vi "MR-Main.vi"() -> ()   [LabVIEW 2017]
doc: "The MyRIO MR-Main programme is a debug level operation that allows an authorised, TCP/IP capable controller to simulate customisable cooling events via control of a PWM servo and also transfer of information, including video, temperature and movement values.\nIf not connected to a remote controller, the programme will operate on a fix independent cooling cycle."
uses:
  <vilib>/myRIO/Express VI/Onboard Devices/Accelerometer/Accelerometer Express VI.xnode
  <vilib>/myRIO/Instrument Drivers/Onboard Devices/Accelerometer/vis/Read.vi
  <vilib>/myRIO/Instrument Drivers/Onboard Devices/Accelerometer/Accelerometer.lvlib
  <vilib>/myRIO/Common/Instrument Driver Framework/myRIO v1.0/Accelerometer/typedefs/Accelerometer Channels Enum.ctl
  <vilib>/myRIO/Common/Instrument Driver Framework/myRIO v1.0/Accelerometer/typedefs/Accelerometer Channels List.ctl
  <vilib>/myRIO/Common/Instrument Driver Framework/Utilities/typedefs/Generic FPGA Reference.ctl
  <vilib>/myRIO/Common/Instrument Driver Framework/Utilities/typedefs/myRIO v1.0 Reference.ctl
  <vilib>/myRIO/Common/Instrument Driver Framework/Utilities/typedefs/Hardware Version Enum.ctl
  <vilib>/myRIO/Common/Instrument Driver Framework/Utilities/typedefs/myRIO Generic Hardware Reference.ctl
  <vilib>/myRIO/Instrument Drivers/Onboard Devices/Accelerometer/typedefs/Accelerometer Reference.ctl
  <vilib>/myRIO/Instrument Drivers/Onboard Devices/Accelerometer/vis/myRIO Accelerometer Open.xnode
  <vilib>/myRIO/Common/Instrument Driver Framework/Utilities/vis/Is FPGA Ref Available.vi
  <vilib>/myRIO/Common/Instrument Driver Framework/myRIO v1.0/Accelerometer/vis/myRIO v1.1 Open Accelerometer.vi
  <vilib>/userdefined/High Color/nirio_resource_hc.ctl
  <vilib>/myRIO/Express VI/Onboard IO/AI/AI Express VI.xnode
  <vilib>/myRIO/Instrument Drivers/Onboard IO/AI/vis/Read.vi
  <vilib>/myRIO/Instrument Drivers/Onboard IO/AI/AI.lvlib
  <vilib>/myRIO/Common/Instrument Driver Framework/Utilities/typedefs/Analog Scaling Constants.ctl
  <vilib>/myRIO/Common/Instrument Driver Framework/Utilities/typedefs/Analog Scaling Constants List.ctl
  <vilib>/myRIO/Common/Instrument Driver Framework/myRIO v1.0/AI/typedefs/AI Channels Enum.ctl
  <vilib>/myRIO/Common/Instrument Driver Framework/myRIO v1.0/AI/typedefs/AI Channels List.ctl
  <vilib>/myRIO/Instrument Drivers/Onboard IO/AI/typedefs/AI Reference.ctl
  <vilib>/myRIO/Instrument Drivers/Onboard IO/AI/vis/myRIO AI Open.xnode
  <vilib>/myRIO/Common/Instrument Driver Framework/myRIO v1.0/AI/vis/myRIO v1.1 Open AI.vi
  <vilib>/myRIO/Express VI/Onboard Devices/LED/LED Express VI.xnode
  <vilib>/myRIO/Instrument Drivers/Onboard IO/DIO/vis/Write.vi
  <vilib>/myRIO/Instrument Drivers/Onboard IO/DIO/DIO.lvlib
  <vilib>/myRIO/Common/Instrument Driver Framework/myRIO v1.0/DIO/typedefs/DIO Channels Enum.ctl
  <vilib>/myRIO/Common/Instrument Driver Framework/myRIO v1.0/DIO/typedefs/DIO Channels List.ctl
  <vilib>/myRIO/Instrument Drivers/Onboard IO/DIO/typedefs/DIO Reference.ctl
  <vilib>/myRIO/Instrument Drivers/Onboard IO/DIO/vis/myRIO DIO Open.xnode
  <vilib>/myRIO/Common/Instrument Driver Framework/myRIO v1.0/DIO/vis/myRIO v1.1 Open DIO.vi
  <vilib>/myRIO/Express VI/Onboard IO/PWM/PWM Express VI.xnode
  <vilib>/myRIO/Instrument Drivers/Onboard IO/PWM/vis/Set Duty Cycle and Frequency.vi
  <vilib>/myRIO/Instrument Drivers/Onboard IO/PWM/PWM.lvlib
  <vilib>/myRIO/Instrument Drivers/Onboard IO/PWM/typedefs/PWM Configuration.ctl
  <vilib>/myRIO/Common/Instrument Driver Framework/myRIO v1.0/PWM/typedefs/PWM Channels Enum.ctl
  <vilib>/myRIO/Instrument Drivers/Onboard IO/PWM/typedefs/PWM Reference.ctl
  <vilib>/myRIO/Instrument Drivers/Onboard IO/PWM/vis/myRIO PWM Open.xnode
  <vilib>/myRIO/Common/Instrument Driver Framework/myRIO v1.0/PWM/vis/myRIO v1.1 Open PWM.vi
  <vilib>/myRIO/Express VI/Onboard Devices/Button/Button Express VI.xnode
  <vilib>/myRIO/Instrument Drivers/Onboard IO/DIO/vis/Read.vi
  <vilib>/myRIO/Instrument Drivers/Utilities/Utilities.lvlib
  <vilib>/vision/driver/NI_Vision_Acquisition_Software.lvlib
  <vilib>/userdefined/High Color/IMAQdx.ctl
  <resource>/objmgr/imaqdx.rc
panel:
  in  "Timeout Control":i32=30
  in  "Turn Off Counter":i32=10
  out "Turn Off Timer":timestamp format="%<%H:%M:%S>T"
  in  "Destruction Counter":i32=10
  in  "VideoMode":u32
  in  "Session In":T1
  out "Timeout":bool
  out "Timeout":timestamp format="%<%H:%M:%S>T"
  out "Scheduler":bool
  out "Destroyed":bool
  out "Destruction Timer":timestamp format="%<%H:%M:%S>T"
  in  "Disconnect":bool
  in  "Status Value":u8=1
  out "Local\nRequest":bool
  out "Movement\nDetected":bool
  out "Movement Event Array":bool[](array[boolean])
  in  "Lower\nTolerance":dbl=1.0 format="%#.3g"
  in  "Upper\nTolerance":dbl=1.0 format="%#.13g"
  out "Cooling Event Array":bool[](array[boolean])
  out "System Time":timestamp format="%<%H:%M:%S>T"
  in  "Cooling 4 Off":timestamp format="%<%H:%M:%S>T"
  in  "Cooling 4 On":timestamp format="%<%H:%M:%S>T"
  in  "Cooling 3 Off":timestamp format="%<%H:%M:%S>T"
  in  "Cooling 3 On":timestamp format="%<%H:%M:%S>T"
  in  "Cooling 2 Off":timestamp format="%<%H:%M:%S>T"
  in  "Cooling 2 On":timestamp format="%<%H:%M:%S>T"
  in  "Cooling 1 Off":timestamp format="%<%H:%M:%S>T"
  in  "Cooling 1 On":timestamp format="%<%H:%M:%S>T"
  out "Master Controller":bool
  out "Local Controller":bool
  out "Emergency Cooling":bool
  out "Initial Z":dbl=1.0 format="%#_13g"
  out "Initial Y":dbl=1.0 format="%#_13g"
  out "Initial X":dbl=1.0 format="%#_13g"
  in  "Emergency Temp (C)":u32=26
  out "source":string
  out "status":bool
  out "code":i32
  out "Net Error Code":i32
  out "Temp (C)":dbl format="%#.1g"
  out "Scheduled Cooling":bool
  out "Cooling 4":bool
  out "Cooling 3":bool
  out "Cooling 2":bool
  out "Cooling 1":bool
  out "Waveform Chart":T2(graph)
  out "String Length":i32
  out "Bytes Written":i32
  in  "Stop":bool
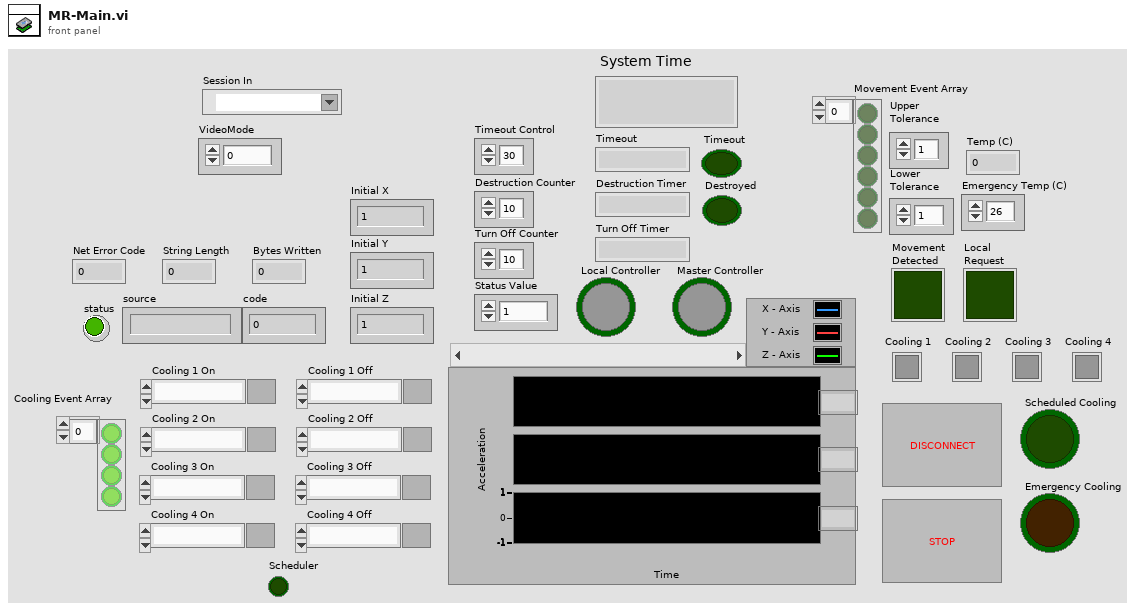
[diagram p1: front panel]
types:
  T1 = typedef "IMAQdx.ctl" = refnum<k21>
  T2 = cluster{"X-Axis":dbl, "Y-Axis":dbl, "Z-Axis":dbl}
  T3 = typedef "DIO.lvlib/DIO Reference.ctl" = cluster{"myRIO Reference":T4, "DIO Channels List":T8}
  T4 = typedef "myRIO Generic Hardware Reference.ctl" = cluster{"myRIO Model":T5, "myRIO Hardware Reference":T6}
  T5 = typedef "Hardware Version Enum.ctl" = enum16{"Unknown", "myRIO-1900", "myRIO-1950", "roboRIO", "NI ELVIS RIO CM"}
  T6 = typedef "myRIO v1.0 Reference.ctl" = cluster{"Generic FPGA Reference":T7, "Allow multiple opens":bool}
  T7 = typedef "Generic FPGA Reference.ctl" = refnum<k20>
  T8 = typedef "DIO Channels List.ctl" = T9[]
  T9 = typedef "DIO Channels Enum.ctl" = enum16{"Not Connected", "C/DIO0", "C/DIO1", "C/DIO2", "C/DIO3", "C/DIO4", "C/DIO5", "C/DIO6", "C/DIO7", "A/DIO0", "A/DIO1", "A/DIO2", "A/DIO3", "A/DIO4", "A/DIO5", "A/DIO6", "A/DIO7", "A/DIO8", "A/DIO9", "A/DIO10", "A/DIO11", "A/DIO12", "A/DIO13", "A/DIO14", "A/DIO15", "B/DIO0", "B/DIO1", "B/DIO2", "B/DIO3", "B/DIO4", "B/DIO5", "B/DIO6", "B/DIO7", "B/DIO8", "B/DIO9", "B/DIO10", "B/DIO11", "B/DIO12", "B/DIO13", "B/DIO14", "B/DIO15", "LED0", "LED1", "LED2", "LED3", "Button0", "DIO/DIO0", "DIO/DIO1", "DIO/DIO2", "DIO/DIO3", "DIO/DIO4", "DIO/DIO5", "DIO/DIO6", "DIO/DIO7", "DIO/DIO8", "DIO/DIO9", "SPI/CS0", "SPI/CS1", "SPI/CS2", "SPI/CS3", "LED RADIO (Green)", "LED RADIO (Red)", "LED COMM (Green)", "LED COMM (Red)", "LED MODE (Green)", "LED MODE (Red)"}
  T10 = typedef "nirio_resource_hc.ctl" = tag
  T11 = typedef "AI.lvlib/AI Reference.ctl" = cluster{"myRIO Reference":T4, "AI Channels List":T12, "AI Scaling Constants List":T14}
  T12 = typedef "AI Channels List.ctl" = T13[]
  T13 = typedef "AI Channels Enum.ctl" = enum16{"Not Connected", "AudioIn/Left", "AudioIn/Right", "C/AI0", "C/AI1", "A/AI0", "A/AI1", "A/AI2", "A/AI3", "B/AI0", "B/AI1", "B/AI2", "B/AI3", "AI/AI0", "AI/AI1", "AI/AI2", "AI/AI3"}
  T14 = typedef "Analog Scaling Constants List.ctl" = T15[]
  T15 = typedef "Analog Scaling Constants.ctl" = cluster{"LSB Weight (Volts)":dbl, "Offset (Volts)":dbl, "Signed?":bool}
  T16 = typedef "PWM.lvlib/PWM Reference.ctl" = cluster{"myRIO Reference":T4, "PWM Channels Enum":T17, "PWM Configuration":T18}
  T17 = typedef "PWM Channels Enum.ctl" = enum16{"Not Connected", "C/PWM0", "C/PWM1", "A/PWM0", "A/PWM1", "A/PWM2", "B/PWM0", "B/PWM1", "B/PWM2", "PWM/PWM0", "PWM/PWM1", "PWM/PWM2", "PWM/PWM3", "PWM/PWM4", "PWM/PWM5", "PWM/PWM6", "PWM/PWM7", "PWM/PWM8", "PWM/PWM9"}
  T18 = typedef "PWM.lvlib/PWM Configuration.ctl" = cluster{"Frequency":dbl, "Duty Cycle":dbl}
  T19 = typedef "Accelerometer.lvlib/Accelerometer Reference.ctl" = cluster{"myRIO Reference":T4, "Accelerometer Channels List":T20, "LSB Weight":dbl}
  T20 = typedef "Accelerometer Channels List.ctl" = T21[]
  T21 = typedef "Accelerometer Channels Enum.ctl" = enum16{"Not Connected", "X-Axis", "Y-Axis", "Z-Axis"}
  T22 = typedef "Image Type" = u32
  T23 = typedef "IMAQ Image.ctl" = refnum<image>
  T24 = cluster{dbl, dbl, dbl, dbl, bool, u8, "Status Value":u8}
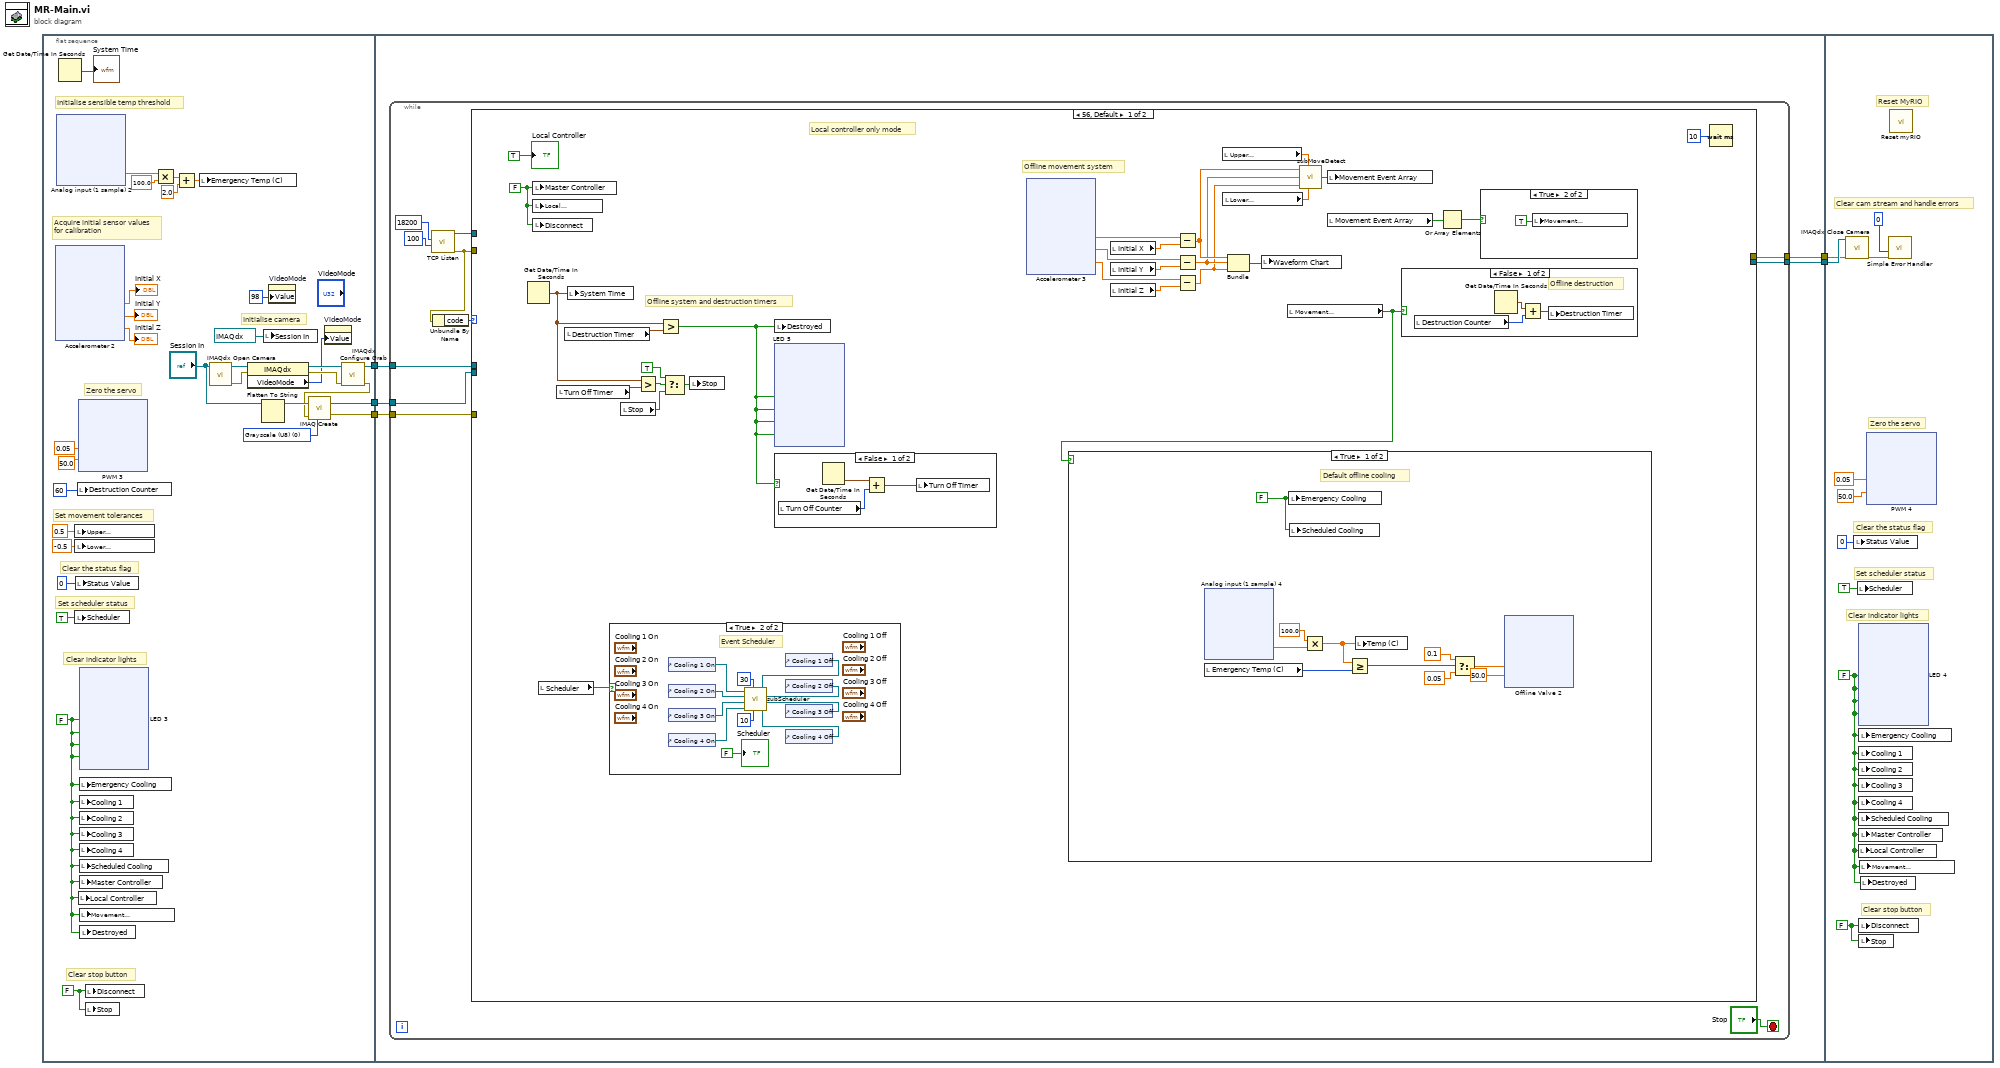
[diagram p0: block diagram]
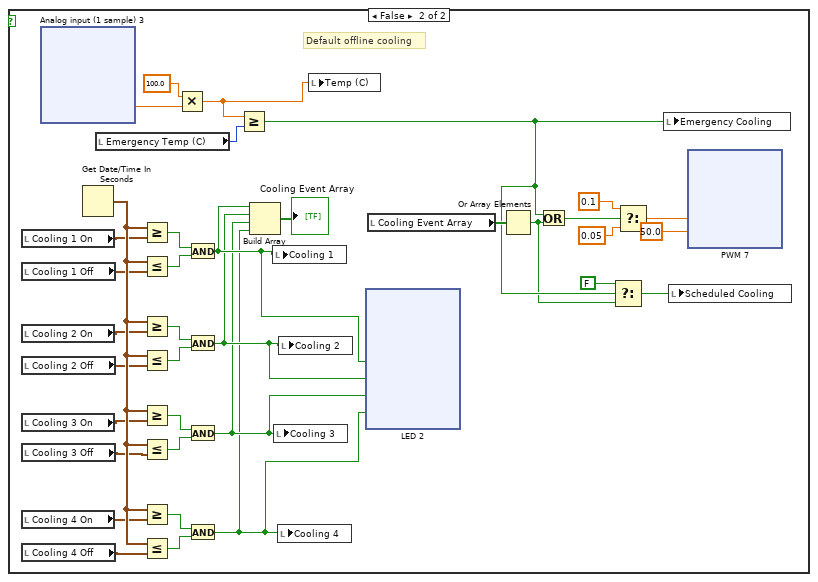
[diagram p3: hidden frame]
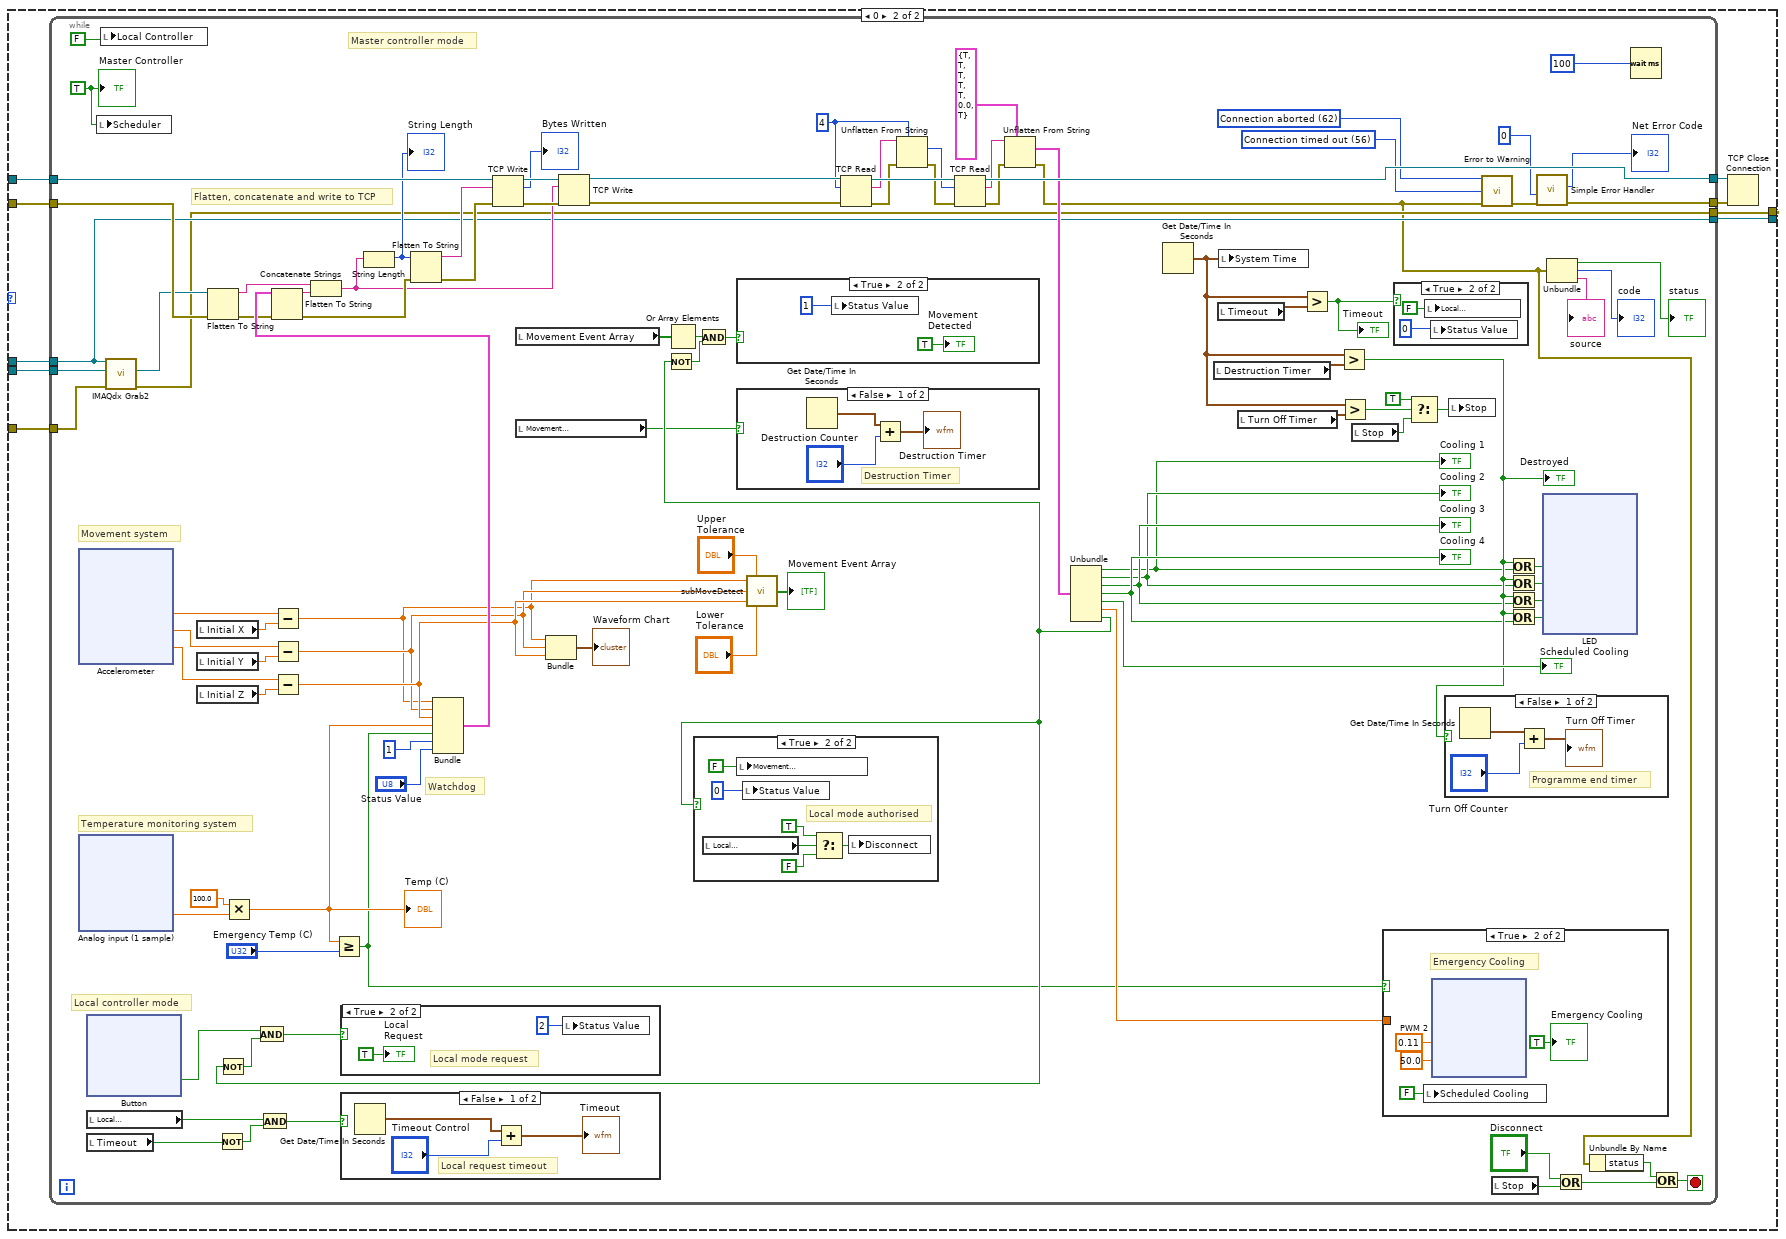
[diagram p7: hidden frame]
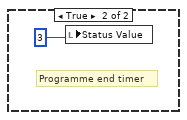
[diagram p8: hidden frame]
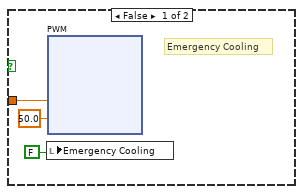
[diagram p15: hidden frame]
diagram:
  n1 = flat-sequence {
    tunnel: [w20] -> w5
    tunnel: [w19] -> w4
    tunnel: [w10] -> w1
    tunnel: w5 -> [w191]
    tunnel: w4 -> [w190]
    tunnel: [w189] -> w3
    tunnel: [w188] -> w2
    tunnel: w1 -> [w187]
    tunnel: w3 -> [w919]
    tunnel: w2 -> [w918]
    frame #0 {
      w16 = T22 0 items=["Grayscale (U8)", "Grayscale (I16)", "Grayscale (SGL)", "Complex (CSG)", "RGB (U32)", "HSL (U32)", "RGB (U64)", "Grayscale (U16)"] ("Image Type")
      w9 = FALSE
      w24 = FALSE
      # "Set scheduler status"
      # "Clear the status flag"
      # "Initialise camera"
      # "Clear indicator lights"
      # "Set movement tolerances"
      # "Zero the servo"
      # "Initialise sensible temp threshold"
      # "Acquire initial sensor values\nfor calibration"
      # "Clear stop button"
      n2 = xnode "Accelerometer 2"() -> ("X-Axis"=→"Initial X":dbl, "Y-Axis"=→"Initial Y":dbl, "Z-Axis"=→"Initial Z":dbl)  [unwired: 1 in, 1 out]
      n3 = xnode "Analog input (1 sample) 2"() -> ("A/AI3 (Pin 9)"=w29:dbl)  [unwired: 1 in, 1 out]
      n4 = Get Date/Time In Seconds() -> (seconds since 1Jan1904=→"System Time":timestamp)
      n5 = local write "Upper\nTolerance"(0.5 ("Upper\nTolerance")) -> ()
      n6 = local write "Lower\nTolerance"(-0.5 ("Lower\nTolerance 2")) -> ()
      n7 = local write "Scheduler"(TRUE) -> ()
      n8 = local write "Status Value"(u8 0 ("Request Value")) -> ()
      n9 = local write "Destruction Counter"(60) -> ()
      n10 = xnode "PWM 3"("Duty Cycle"=0.05, "Frequency [Hz]"=50.0) -> ()  [unwired: 1 in, 1 out]
      n11 = local write "Local Controller"(w9) -> ()
      n12 = xnode "LED 3"("LED0"=w9, "LED1"=w9, "LED2"=w9, "LED3"=w9) -> ()  [unwired: 1 in, 1 out]
      n13 = local write "Emergency Cooling"(w9) -> ()
      n14 = local write "Cooling 1"(w9) -> ()
      n15 = local write "Cooling 2"(w9) -> ()
      n16 = local write "Cooling 3"(w9) -> ()
      n17 = local write "Cooling 4"(w9) -> ()
      n18 = local write "Scheduled Cooling"(w9) -> ()
      n19 = local write "Master Controller"(w9) -> ()
      n20 = local write "Movement\nDetected"(w9) -> ()
      n21 = local write "Destroyed"(w9) -> ()
      n22 = local write "Disconnect"(w24) -> ()
      n23 = local write "Stop"(w24) -> ()
      n24 = Multiply(x=w29, y=100.0) -> (x*y=w30:dbl)
      n25 = Add(x=w30, y=2.0) -> (x+y=w31:dbl)
      n26 = local write "Emergency Temp (C)"(w31) -> ()
      n27 = call <vilib>:"IMAQdx Open Camera.vi"("Session In"="Session In") -> ("error out"=w13:errorcluster, "Session Out"=w15:T1)  [unwired: 2 in, 7 out]
      n28 = property class="IMAQdx"(reference=w15, error in=w13) -> (reference out=w14:T1, error out=w12:errorcluster, "VideoMode"=w8:u32)
      n29 = Flatten To String(anything="Session In") -> (data string=w17:string)  [unwired: 3 in, 2 out]
      n30 = local write "Session In"(T1 "cam0" ("Session In")) -> ()
      n31 = property on="VideoMode" class="DigNum (strict)"("Value"=u32 98 ("VideoMode")) -> ()  [unwired: 2 in, 2 out]
      n32 = property on="VideoMode" class="DigNum (strict)"("Value"=w8) -> ()  [unwired: 2 in, 2 out]
      n33 = call <vilib>:"IMAQdx Configure Grab.vi"("error in"=w12, "Session In"=w14) -> ("error out"=w11:errorcluster, "Session Out"=w20:T1)  [unwired: 2 in, 6 out]
      n34 = call "IMAQ Create"("Image Name"=w17, "Image Type"=w16, "error in (no error)"=w11) -> ("New Image"=w19:T23, "error out"=w10:errorcluster)  [unwired: 2 in]
    }
    frame #1 {
      n35 = while {
        tunnel: w191 -> [w196]
        tunnel: w190 -> [w195]
        tunnel: [w194] -> w189
        tunnel: [w193] -> w188
        tunnel: w187 -> [w192]
        stop <- "Stop" stop-if-true
        n36 = call <vilib>:"TCP Listen.vi"("timeout ms (wait forever: -1)"=100, "port"=u16 18200 ("timeout ms (wait forever: -1)")) -> ("error out"=w198:errorcluster, "connection ID"=w201:refnum<k5>)  [unwired: 2 in, 6 out]
        n37 = Unbundle By Name(w198) -> ("code"=w197:i32)
        n38 = case shown="56, Default" w197 {
          tunnel: w201 -> [_ w562]
          tunnel: w198 -> [_ w561]
          tunnel: w196 -> [_ w558]
          tunnel: w195 -> [_ w557]
          tunnel: [_ w556] -> w194
          tunnel: [_ w555] -> w193
          tunnel: w192 -> [_ w554]
          frame 56, Default {
            w223 = FALSE
            # "Offline system and destruction timers"
            # "Offline movement system"
            # "Local controller only mode"
            n39 = Get Date/Time In Seconds() -> (seconds since 1Jan1904=w208:timestamp)
            n40 = local write "Master Controller"(w223) -> ()
            n41 = local write "Local\nRequest"(w223) -> ()
            n42 = local write "Disconnect"(w223) -> ()
            n43 = local read "Scheduler"() -> (w212:bool)
            n44 = local read "Turn Off Timer"() -> (w209:timestamp)
            n45 = local read "Destruction Timer"() -> (w214:timestamp)
            n46 = local write "System Time"(w208) -> ()
            n47 = case shown="True" w212 {
              frame False {
              }
              frame True {
                # "Event Scheduler"
                n48 = control-ref of="Cooling 1 On"() -> (w503:refnum<vi>)
                n49 = control-ref of="Cooling 2 On"() -> (w502:refnum<vi>)
                n50 = control-ref of="Cooling 3 On"() -> (w501:refnum<vi>)
                n51 = control-ref of="Cooling 4 On"() -> (w500:refnum<vi>)
                n52 = control-ref of="Cooling 1 Off"() -> (w507:refnum<vi>)
                n53 = control-ref of="Cooling 2 Off"() -> (w505:refnum<vi>)
                n54 = control-ref of="Cooling 3 Off"() -> (w504:refnum<vi>)
                n55 = control-ref of="Cooling 4 Off"() -> (w506:refnum<vi>)
                n56 = call "subScheduler.vi"("Cooling 4 Off"=w506, "Cooling 3 Off"=w504, "Cooling 2 Off"=w505, "Cooling 1 Off"=w507, "Deactivate Offset"=10, "Activate Offset"=30, "Cooling 4 On"=w500, "Cooling 3 On"=w501, "Cooling 2 On"=w502, "Cooling 1 On"=w503) -> ()
                "Scheduler" <- FALSE
              }
            }
            n57 = local read "Stop"() -> (w204:bool)
            n58 = Greater?(x=w208, y=w209) -> (0:w206:bool)
            n59 = Greater?(x=w208, y=w214) -> (0:w207:bool)
            n60 = Select(t=TRUE, s=w206, f=w204) -> (s? t:f=w205:bool)
            n61 = local write "Stop"(w205) -> ()
            n62 = case shown="False" w207 {
              frame False {
                n63 = local read "Turn Off Counter"() -> (w232:i32)
                n64 = Get Date/Time In Seconds() -> (seconds since 1Jan1904=w233:timestamp)
                n65 = Add(x=w233, y=w232) -> (x+y=w231:timestamp)
                n66 = local write "Turn Off Timer"(w231) -> ()
              }
              frame True {
              }
            }
            n67 = local write "Destroyed"(w207) -> ()
            n68 = xnode "LED 5"("LED0"=w207, "LED1"=w207, "LED2"=w207, "LED3"=w207) -> ()  [unwired: 1 in, 1 out]
            n69 = xnode "Accelerometer 3"() -> ("X-Axis"=w226:dbl, "Y-Axis"=w228:dbl, "Z-Axis"=w230:dbl)  [unwired: 1 in, 1 out]
            n70 = local read "Initial X"() -> (w225:dbl)
            n71 = local read "Initial Y"() -> (w227:dbl)
            n72 = local read "Initial Z"() -> (w229:dbl)
            n73 = Subtract(x=w226, y=w225) -> (x-y=w221:dbl)
            n74 = Subtract(x=w228, y=w227) -> (x-y=w220:dbl)
            n75 = Subtract(x=w230, y=w229) -> (x-y=w219:dbl)
            n76 = local read "Upper\nTolerance"() -> (w217:dbl)
            n77 = local read "Lower\nTolerance"() -> (w218:dbl)
            n78 = Bundle(w221, w220, w219) -> (w224:cluster{dbl, dbl, dbl})  [unwired: 1 in]
            n79 = local write "Waveform Chart"(w224) -> ()
            n80 = local read "Movement\nDetected"() -> (w211:bool)
            n81 = case shown="True" w211 {
              frame True {
                w281 = FALSE
                # "Default offline cooling"
                n82 = xnode "Analog input (1 sample) 4"() -> ("A/AI3 (Pin 9)"=w276:dbl)  [unwired: 1 in, 1 out]
                n83 = local read "Emergency Temp (C)"() -> (w274:u32)
                n84 = local write "Emergency Cooling"(w281) -> ()
                n85 = local write "Scheduled Cooling"(w281) -> ()
                n86 = Multiply(x=100.0, y=w276) -> (x*y=w273:dbl)
                n87 = Greater Or Equal?(x=w273, y=w274) -> (x >= y?=w272:bool)
                n88 = local write "Temp (C)"(w273) -> ()
                n89 = Select(t=0.1, s=w272, f=0.05) -> (s? t:f=w277:dbl)
                n90 = xnode "Offline Valve 2"("Duty Cycle"=w277, "Frequency [Hz]"=50.0) -> ()  [unwired: 1 in, 1 out]
              }
              frame False {
                # "Default offline cooling"
                n91 = local read "Cooling 1 On"() -> (w380:timestamp)
                n92 = local read "Cooling 1 Off"() -> (w379:timestamp)
                n93 = local read "Cooling 2 On"() -> (w378:timestamp)
                n94 = local read "Cooling 2 Off"() -> (w377:timestamp)
                n95 = local read "Cooling 3 On"() -> (w376:timestamp)
                n96 = local read "Cooling 3 Off"() -> (w375:timestamp)
                n97 = local read "Cooling 4 On"() -> (w374:timestamp)
                n98 = local read "Cooling 4 Off"() -> (w373:timestamp)
                n99 = xnode "Analog input (1 sample) 3"() -> ("A/AI3 (Pin 9)"=w364:dbl)  [unwired: 1 in, 1 out]
                n100 = Get Date/Time In Seconds() -> (seconds since 1Jan1904=w381:timestamp)
                n101 = local read "Emergency Temp (C)"() -> (w363:u32)
                n102 = Greater Or Equal?(x=w381, y=w380) -> (x >= y?=w388:bool)
                n103 = Less Or Equal?(x=w381, y=w379) -> (x <= y?=w389:bool)
                n104 = Greater Or Equal?(x=w381, y=w378) -> (x >= y?=w387:bool)
                n105 = Less Or Equal?(x=w381, y=w377) -> (x <= y?=w386:bool)
                n106 = Greater Or Equal?(x=w381, y=w376) -> (x >= y?=w384:bool)
                n107 = Less Or Equal?(x=w381, y=w375) -> (x <= y?=w385:bool)
                n108 = Greater Or Equal?(x=w381, y=w374) -> (x >= y?=w383:bool)
                n109 = Less Or Equal?(x=w381, y=w373) -> (x <= y?=w382:bool)
                n110 = Multiply(x=100.0, y=w364) -> (x*y=w362:dbl)
                n111 = And(x=w388, y=w389) -> (x .and. y?=w369:bool)
                n112 = And(x=w387, y=w386) -> (x .and. y?=w368:bool)
                n113 = And(x=w384, y=w385) -> (x .and. y?=w367:bool)
                n114 = And(x=w383, y=w382) -> (x .and. y?=w366:bool)
                n115 = Greater Or Equal?(x=w362, y=w363) -> (x >= y?=w359:bool)
                n116 = Build Array(w369, w368, w367, w366) -> (→"Cooling Event Array":bool[])
                n117 = local write "Cooling 1"(w369) -> ()
                n118 = local write "Cooling 3"(w367) -> ()
                n119 = local write "Cooling 4"(w366) -> ()
                n120 = local write "Cooling 2"(w368) -> ()
                n121 = local write "Temp (C)"(w362) -> ()
                n122 = xnode "LED 2"("LED0"=w369, "LED1"=w368, "LED2"=w367, "LED3"=w366) -> ()  [unwired: 1 in, 1 out]
                n123 = local read "Cooling Event Array"() -> (w371:bool[])
                n124 = Or Array Elements(Boolean array=w371) -> (logical OR=w358:bool)
                n125 = Or(x=w359, y=w358) -> (x .or. y?=w361:bool)
                n126 = Select(t=FALSE, s=w359, f=w358) -> (s? t:f=w356:bool)
                n127 = Select(t=0.1, s=w361, f=0.05) -> (s? t:f=w354:dbl)
                n128 = local write "Emergency Cooling"(w359) -> ()
                n129 = local write "Scheduled Cooling"(w356) -> ()
                n130 = xnode "PWM 7"("Duty Cycle"=w354, "Frequency [Hz]"=50.0) -> ()  [unwired: 1 in, 1 out]
              }
            }
            n131 = call "subMoveDetect.vi"("X"=w221, "Upper\nTolerance"=w217, "Y"=w220, "Z"=w219, "Lower\nTolerance"=w218) -> ("Movement Event Array"=w222:bool[])
            n132 = local write "Movement Event Array"(w222) -> ()
            n133 = local read "Movement Event Array"() -> (w216:bool[])
            n134 = case shown="False" w211 {
              frame False {
                # "Offline destruction"
                n135 = local read "Destruction Counter"() -> (w512:i32)
                n136 = Get Date/Time In Seconds() -> (seconds since 1Jan1904=w514:timestamp)
                n137 = Add(x=w514, y=w512) -> (x+y=w513:timestamp)
                n138 = local write "Destruction Timer"(w513) -> ()
              }
              frame True {
              }
            }
            n139 = Or Array Elements(Boolean array=w216) -> (logical OR=w215:bool)
            n140 = case shown="True" w215 {
              frame False {
              }
              frame True {
                n141 = local write "Movement\nDetected"(TRUE) -> ()
              }
            }
            n142 = Wait (ms)(milliseconds to wait=u32 10) -> ()  [unwired: 1 out]
            "Local Controller" <- TRUE
          }
          frame 0 {
            n143 = while {
              tunnel: w562 -> [w662]
              tunnel: w561 -> [w581]
              tunnel: [w604] -> w560
              tunnel: [w656] -> w559
              tunnel: w558 -> [w578]
              tunnel: w557 -> [w579]
              tunnel: [w578] -> w556
              tunnel: [w573] -> w555
              tunnel: w554 -> [w577]
              stop <- w661 stop-if-true
              w592 = TRUE
              w650 = 56 items=["No Error", "Argument Error", "Memory Full", "Out of Zone", "End of File", "File Already Open", "Generic File IO Error", "File Not Found", "File Permission Error", "Disk Full", "Duplicate Path", "Too Many Files Open", "Not Enabled", "Resource File Not Found", "Cannot Add Resource", "Resource Not Found", "Image Not Found", "Image Memory Error", "Pen Does Not Exist", "Config Bad Type", "Config Token Not Found", "Config Parse Error", "Config Memory Error", "Bad External Code Format", "Bad External Code Offset", "External Code Not Present", "Null Window", "Destroy Window Mixup", "Null Menu", "Print Aborted", "Bad Print Record", "Print Driver Error", "Windows Error During Print", "Memory Error During Print", "Print Dialog Error", "Generic Print Error", "Invalid Device Refnum", "Device Not Found", "Device Parameter Error", "Device Unit Error", "Can't Open Device", "Device Call Aborted", "Generic Error", "Cancelled By User", "Object ID Too Low", "Object ID Too High", "Object Not In Heap", "Unknown Heap", "Bad DefProc ID", "DefProc Not In Table", "Message Out Of Range", "Null Method", "Unknown Message", "Manager Call Not Supported", "Bad address", "Connection In progress", "Connection timed out", "Connection is already in progress", "Network attribute not supported", "Network error", "Address in use", "System out of memory", "Connection aborted", "Connection refused", "Connection is not connected", "Connection is already connected", "Connection closed", "Initialize error (interapplication manager)", "Bad occurrence", "Wait on unbound occurrence handler", "Occurrence queue overflow", "Bad path", "Semaphore not signaled", "Unrecognized type (interapplication manager)"] ("3rd Error to Convert")
              w651 = 62 items=["No Error", "Argument Error", "Memory Full", "Out of Zone", "End of File", "File Already Open", "Generic File IO Error", "File Not Found", "File Permission Error", "Disk Full", "Duplicate Path", "Too Many Files Open", "Not Enabled", "Resource File Not Found", "Cannot Add Resource", "Resource Not Found", "Image Not Found", "Image Memory Error", "Pen Does Not Exist", "Config Bad Type", "Config Token Not Found", "Config Parse Error", "Config Memory Error", "Bad External Code Format", "Bad External Code Offset", "External Code Not Present", "Null Window", "Destroy Window Mixup", "Null Menu", "Print Aborted", "Bad Print Record", "Print Driver Error", "Windows Error During Print", "Memory Error During Print", "Print Dialog Error", "Generic Print Error", "Invalid Device Refnum", "Device Not Found", "Device Parameter Error", "Device Unit Error", "Can't Open Device", "Device Call Aborted", "Generic Error", "Cancelled By User", "Object ID Too Low", "Object ID Too High", "Object Not In Heap", "Unknown Heap", "Bad DefProc ID", "DefProc Not In Table", "Message Out Of Range", "Null Method", "Unknown Message", "Manager Call Not Supported", "Bad address", "Connection In progress", "Connection timed out", "Connection is already in progress", "Network attribute not supported", "Network error", "Address in use", "System out of memory", "Connection aborted", "Connection refused", "Connection is not connected", "Connection is already connected", "Connection closed", "Initialize error (interapplication manager)", "Bad occurrence", "Wait on unbound occurrence handler", "Occurrence queue overflow", "Bad path", "Semaphore not signaled", "Unrecognized type (interapplication manager)"] ("1st Error to Convert")
              w630 = 4 ("bytes to read")
              # "Master controller mode"
              # "Movement system"
              # "Temperature monitoring system"
              # "Watchdog"
              # "Flatten, concatenate and write to TCP"
              # "Local controller mode"
              n144 = xnode "Accelerometer"() -> ("X-Axis"=w640:dbl, "Y-Axis"=w641:dbl, "Z-Axis"=w653:dbl)  [unwired: 1 in, 1 out]
              n145 = xnode "Analog input (1 sample)"() -> ("A/AI3 (Pin 9)"=w660:dbl)  [unwired: 1 in, 1 out]
              n146 = xnode "Button"() -> ("Value"=w611:bool)  [unwired: 1 in, 1 out]
              n147 = local read "Local\nRequest"() -> (w586:bool)
              n148 = local read "Timeout"() -> (w583:bool)
              n149 = local write "Scheduler"(w592) -> ()
              n150 = local write "Local Controller"(FALSE) -> ()
              n151 = call <vilib>:"IMAQdx Grab2.vi"("error in"=w577, "Image In"=w579, "Session In"=w578) -> ("error out"=w573:errorcluster, "Image Out"=w580:T23)  [unwired: 5 in, 2 out]
              n152 = local read "Initial X"() -> (w637:dbl)
              n153 = local read "Initial Y"() -> (w638:dbl)
              n154 = local read "Initial Z"() -> (w639:dbl)
              n155 = Flatten To String(anything=w580, error in (no error)=w581) -> (data string=w617:string, error out=w625:errorcluster)  [unwired: 2 in, 1 out]
              n156 = Not(x=w583) -> (.not. x?=w585:bool)
              n157 = Multiply(x=100.0, y=w660) -> (x*y=w649:dbl)
              "Temp (C)" <- w649
              n158 = And(x=w586, y=w585) -> (x .and. y?=w584:bool)
              n159 = Subtract(x=w640, y=w637) -> (x-y=w596:dbl)
              n160 = Subtract(x=w641, y=w638) -> (x-y=w597:dbl)
              n161 = Subtract(x=w653, y=w639) -> (x-y=w598:dbl)
              n162 = Greater Or Equal?(x=w649, y="Emergency Temp (C)") -> (x >= y?=w603:bool)
              n163 = case shown="False" w584 {
                frame False {
                  # "Local request timeout"
                  n164 = Get Date/Time In Seconds() -> (seconds since 1Jan1904=w673:timestamp)
                  n165 = Add(x=w673, y="Timeout Control") -> (x+y=→"Timeout":timestamp)
                }
                frame True {
                  # "Local request timeout"
                }
              }
              n166 = Bundle(w596, w597, w598, w649, w603, u8 1, "Status Value"="Status Value") -> (w634:T24)  [unwired: 1 in]
              n167 = Flatten To String(anything=w634, error in (no error)=w625) -> (data string=w619:string, error out=w624:errorcluster)  [unwired: 2 in, 1 out]
              n168 = Concatenate Strings(w617, w619) -> (w618:string)
              n169 = String Length(string=w618) -> (length=w633:i32)
              "String Length" <- w633
              n170 = Flatten To String(anything=w633, error in (no error)=w624) -> (data string=w632:string, error out=w623:errorcluster)  [unwired: 2 in, 1 out]
              n171 = TCP Write(connection ID=w662, data in=w632, error in (no error)=w623) -> (connection ID out=w663:refnum<k5>, bytes written=→"Bytes Written":i32, error out=w664:errorcluster)  [unwired: 1 out]
              n172 = local read "Movement Event Array"() -> (w635:bool[])
              n173 = local read "Movement\nDetected"() -> (w599:bool)
              n174 = Bundle(w596, w597, w598) -> (→"Waveform Chart":cluster{dbl, dbl, dbl})  [unwired: 1 in]
              n175 = TCP Write(connection ID=w663, data in=w618, error in (no error)=w664) -> (connection ID out=w658:refnum<k5>, error out=w643:errorcluster)  [unwired: 2 out]
              n176 = Or Array Elements(Boolean array=w635) -> (logical OR=w615:bool)
              n177 = case shown="False" w599 {
                frame False {
                  # "Destruction Timer"
                  n178 = Get Date/Time In Seconds() -> (seconds since 1Jan1904=w677:timestamp)
                  n179 = Add(x=w677, y="Destruction Counter") -> (x+y=→"Destruction Timer":timestamp)
                }
                frame True {
                }
              }
              n180 = call "subMoveDetect.vi"("X"=w596, "Upper\nTolerance"="Upper\nTolerance", "Y"=w597, "Z"=w598, "Lower\nTolerance"="Lower\nTolerance") -> ("Movement Event Array"=→"Movement Event Array":bool[])
              n181 = TCP Read(connection ID=w658, bytes to read=w630, error in (no error)=w643) -> (connection ID out=w657:refnum<k5>, data out=w631:string, error out=w622:errorcluster)  [unwired: 2 out]
              n182 = Unflatten From String(type=w630, binary string=w631, error in (no error)=w622) -> (value=w629:i32, error out=w621:errorcluster)  [unwired: 2 in, 1 out]
              n183 = TCP Read(connection ID=w657, bytes to read=w629, error in (no error)=w621) -> (connection ID out=w656:refnum<k5>, data out=w628:string, error out=w620:errorcluster)  [unwired: 2 out]
              n184 = Unflatten From String(type=cluster{bool, bool, bool, bool, bool, dbl, bool} {TRUE, TRUE, TRUE, TRUE, TRUE, 0.0, TRUE} ("Cluster"), binary string=w628, error in (no error)=w620) -> (value=w627:cluster{bool, bool, bool, bool, bool, dbl, bool}, error out=w567:errorcluster)  [unwired: 2 in, 1 out]
              n185 = Unbundle(w627) -> (w563:bool, w564:bool, w565:bool, w566:bool, →"Scheduled Cooling":bool, w644:dbl, w608:bool)
              "Cooling 1" <- w563
              "Cooling 2" <- w564
              "Cooling 3" <- w565
              "Cooling 4" <- w566
              n186 = Not(x=w608) -> (.not. x?=w612:bool)
              n187 = And(x=w611, y=w612) -> (x .and. y?=w613:bool)
              n188 = case shown="True" w613 {
                frame False {
                  # "Local mode request"
                }
                frame True {
                  # "Local mode request"
                  n189 = local write "Status Value"(u8 2 ("Request Value")) -> ()
                  "Local\nRequest" <- TRUE
                }
              }
              n190 = Not(x=w608) -> (.not. x?=w614:bool)
              n191 = case shown="True" w608 {
                frame False {
                }
                frame True {
                  # "Local mode authorised"
                  n192 = local read "Local\nRequest"() -> (w683:bool)
                  n193 = local write "Movement\nDetected"(FALSE) -> ()
                  n194 = local write "Status Value"(u8 0 ("Request Value")) -> ()
                  n195 = Select(t=TRUE, s=w683, f=FALSE) -> (s? t:f=w680:bool)
                  n196 = local write "Disconnect"(w680) -> ()
                }
              }
              n197 = And(x=w615, y=w614) -> (x .and. y?=w616:bool)
              n198 = case shown="True" w616 {
                frame False {
                }
                frame True {
                  n199 = local write "Status Value"(u8 1 ("Request Value")) -> ()
                  "Movement\nDetected" <- TRUE
                }
              }
              n200 = Get Date/Time In Seconds() -> (seconds since 1Jan1904=w568:timestamp)
              n201 = local read "Destruction Timer"() -> (w600:timestamp)
              n202 = local read "Timeout"() -> (w587:timestamp)
              n203 = local write "System Time"(w568) -> ()
              n204 = local read "Turn Off Timer"() -> (w575:timestamp)
              n205 = Greater?(x=w568, y=w587) -> (0:w582:bool)
              "Timeout" <- w582
              n206 = Greater?(x=w568, y=w600) -> (0:w576:bool)
              "Destroyed" <- w576
              n207 = Greater?(x=w568, y=w575) -> (0:w572:bool)
              n208 = local read "Stop"() -> (w570:bool)
              n209 = case shown="True" w603 {
                tunnel: w644 -> [w690 _]
                frame False {
                  # "Emergency Cooling"
                  n210 = local write "Emergency Cooling"(FALSE) -> ()
                  n211 = xnode "PWM"("Duty Cycle"=w690, "Frequency [Hz]"=50.0) -> ()  [unwired: 1 in, 1 out]
                }
                frame True {
                  # "Emergency Cooling"
                  n212 = local write "Scheduled Cooling"(FALSE) -> ()
                  n213 = xnode "PWM 2"("Duty Cycle"=0.11, "Frequency [Hz]"=50.0) -> ()  [unwired: 1 in, 1 out]
                  "Emergency Cooling" <- TRUE
                }
              }
              n214 = case shown="True" w582 {
                frame False {
                }
                frame True {
                  n215 = local write "Local\nRequest"(FALSE) -> ()
                  n216 = local write "Status Value"(u8 0 ("Request Value")) -> ()
                }
              }
              n217 = Select(t=TRUE, s=w572, f=w570) -> (s? t:f=w569:bool)
              n218 = case shown="False" w576 {
                frame False {
                  # "Programme end timer"
                  n219 = Get Date/Time In Seconds() -> (seconds since 1Jan1904=w668:timestamp)
                  n220 = Add(x=w668, y="Turn Off Counter") -> (x+y=→"Turn Off Timer":timestamp)
                }
                frame True {
                  # "Programme end timer"
                  n221 = local write "Status Value"(u8 3 ("Request Value")) -> ()
                }
              }
              n222 = local write "Stop"(w569) -> ()
              n223 = call <vilib>:"Error to Warning.vi"("1st Error to Convert"=w651, "3rd Error to Convert"=w650, "error in"=w567) -> ("warning out"=w602:errorcluster)  [unwired: 3 in, 9 out]
              n224 = local read "Stop"() -> (w606:bool)
              n225 = Or(x=w576, y=w563) -> (x .or. y?=w591:bool)
              n226 = Or(x=w576, y=w564) -> (x .or. y?=w590:bool)
              n227 = Or(x=w576, y=w565) -> (x .or. y?=w589:bool)
              n228 = Or(x=w576, y=w566) -> (x .or. y?=w588:bool)
              n229 = call <vilib>:"Simple Error Handler.vi"("type of dialog (OK msg:1)"=0, "error in (no error)"=w602) -> ("code out"=→"Net Error Code":i32, "error out"=w604:errorcluster)  [unwired: 6 out]
              n230 = xnode "LED"("LED0"=w591, "LED1"=w590, "LED2"=w589, "LED3"=w588) -> ()  [unwired: 1 in, 1 out]
              n231 = Unbundle(w567) -> ("status"=→"status":bool, "code"=→"code":i32, "source"=→"source":string)
              n232 = Or(x="Disconnect", y=w606) -> (x .or. y?=w605:bool)
              n233 = Unbundle By Name(w567) -> ("status"=w642:bool)
              n234 = Wait (ms)(milliseconds to wait=u32 100) -> ()  [unwired: 1 out]
              n235 = Or(x=w642, y=w605) -> (x .or. y?=w661:bool)
              "Master Controller" <- w592
            }
            n236 = TCP Close Connection(connection ID=w559, error in (no error)=w560) -> ()  [unwired: 3 out]
          }
        }
      }
    }
    frame #2 {
      w917 = FALSE
      w914 = FALSE
      # "Clear cam stream and handle errors"
      # "Set scheduler status"
      # "Clear the status flag"
      # "Clear indicator lights"
      # "Zero the servo"
      # "Reset MyRIO"
      # "Clear stop button"
      n237 = call <vilib>:"IMAQdx Close Camera.vi"("error in"=w918, "Session In"=w919) -> ("error out"=w916:errorcluster)  [unwired: 9 in]
      n238 = local write "Status Value"(u8 0 ("Request Value")) -> ()
      n239 = local write "Scheduler"(TRUE) -> ()
      n240 = local write "Local Controller"(w917) -> ()
      n241 = xnode "LED 4"("LED0"=w917, "LED1"=w917, "LED2"=w917, "LED3"=w917) -> ()  [unwired: 1 in, 1 out]
      n242 = local write "Emergency Cooling"(w917) -> ()
      n243 = local write "Cooling 1"(w917) -> ()
      n244 = local write "Cooling 2"(w917) -> ()
      n245 = local write "Cooling 3"(w917) -> ()
      n246 = local write "Cooling 4"(w917) -> ()
      n247 = local write "Scheduled Cooling"(w917) -> ()
      n248 = local write "Master Controller"(w917) -> ()
      n249 = local write "Disconnect"(w914) -> ()
      n250 = local write "Stop"(w914) -> ()
      n251 = local write "Movement\nDetected"(w917) -> ()
      n252 = local write "Destroyed"(w917) -> ()
      n253 = xnode "PWM 4"("Duty Cycle"=0.05, "Frequency [Hz]"=50.0) -> ()  [unwired: 1 in, 1 out]
      n254 = call <vilib>:"Simple Error Handler.vi"("type of dialog (OK msg:1)"=0, "error in (no error)"=w916) -> ()  [unwired: 8 out]
      n255 = call <vilib>:"Reset myRIO.vi"() -> ()  [unwired: 11 in, 1 out]
    }
  }
